vi "VisionData.vi"() -> ()   [LabVIEW 2011]
panel:
  in  "AngleWGyro":dbl
  out "VISION NOW":bool
  in  "VisionDataFromcRIO":T1
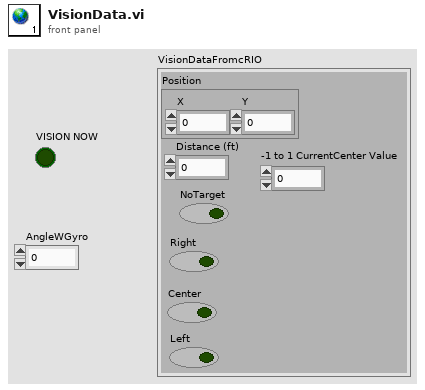
[diagram p1: front panel]
types:
  T1 = cluster{"Position":cluster{"X":dbl, "Y":dbl}, "Distance (ft)":dbl, "NoTarget":bool, "Right":bool, "Center":bool, "Left":bool, "-1 to 1 CurrentCenter Value":dbl}
diagram:
